vi "Update ROI waveform cursor snap selector.vi"(4 "Reset selection to the first element":bool, 8 "error in (no error)":errorcluster) -> (0 "error out":errorcluster)   [LabVIEW 2020]
uses:
  Global variables/gl_Functional Imaging-Global variables.vi
  <userlib>/_OpenG.lib/array/array.llb/Conditional Auto-Indexing Tunnel (String)__ogtk.vi
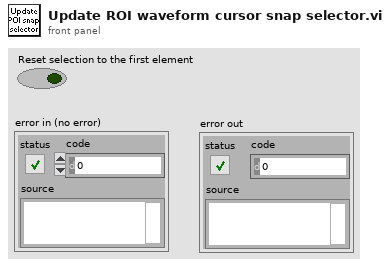
[diagram p1: front panel]
types:
  T1 = typedef "Functional Imging UI Refs.ctl" = cluster{"Menu ref":refnum<k9>, "Image control":refnum<vi>, "VI ref":refnum<vi>, "XGrapher":refnum<vi>, "Smoothing":refnum<vi>, "POI Averaging":refnum<vi>, "Normalize":refnum<vi>, "POI data points in each trial":refnum<vi>, "Channel":refnum<vi>, "Experiment data folder path":refnum<vi>, "[ROI vis]":refnum<vi>, "[Groups] visbl":T2, "Group Name":refnum<vi>, "POI index":refnum<vi>, "Trial No.":refnum<vi>, "Intensity Zoom":refnum<vi>, "Trial Cursor Enabled":refnum<vi>, "Number of Trials (ind 1)":refnum<vi>, "Number of Trials (ind 2)":refnum<vi>, "MiniScans Available":refnum<vi>, "POI Available":refnum<vi>, "Defer graph updates":refnum<vi>, "Waveform selector":refnum<vi>, "#of selected POI":refnum<vi>, "#of selected MiniScans":refnum<vi>, "#of selected groups":refnum<vi>, "Max Z-Projection":refnum<vi>, "Z-Plane Selector":refnum<vi>, "Index of miniscan point to visualise":refnum<vi>, "ROI vis. mode":refnum<vi>, "Total # of points":refnum<vi>, "Index of group clicked on":refnum<vi>, "Pane 1":refnum<vi>, "Pane 2":refnum<vi>, "Pane 3":refnum<vi>, "Pane 4":refnum<vi>, "Pane 5":refnum<vi>, "Pane 6":refnum<vi>, "Deselect all ROI":refnum<vi>, "Deselect all groups":refnum<vi>}
  T2 = typedef "Groups array referecne.ctl" = refnum<vi>
  T3 = typedef "ROI selector array-ROI vis.ctl" = T4[]
  T4 = typedef "Interface-ROI selection cluster.ctl" = cluster{"ROI number":i32, "ROI ID":T5, "Visibility":bool}
  T5 = typedef "ROI ID Enum.ctl" = enum16{"Point", "MiniScan", "Comp. MiniScan", "Rectangle", "Comp. volume", "Arb. plane point", "None"}
  T6 = typedef "Group sel cluster.ctl" = cluster{"Group number":string, "Group Name":string, "Visibility":bool, "Highlight":bool}
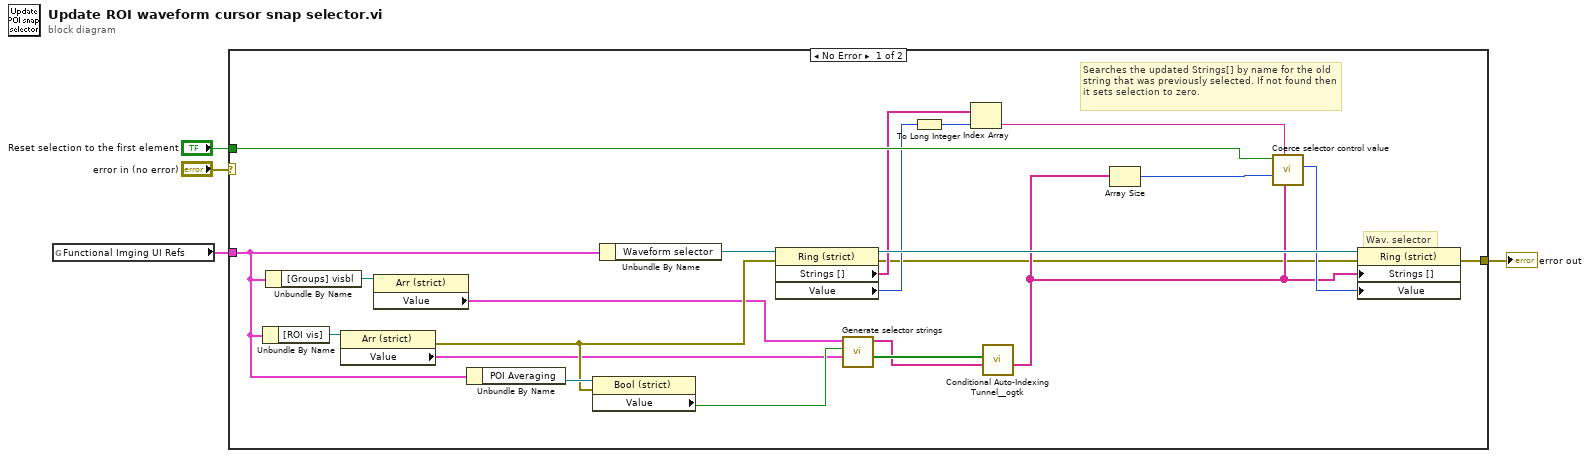
[diagram p0: block diagram]
diagram:
  n1 = global read "gl_Functional Imaging-Global variables.vi" "Functional Imging UI Refs"() -> (w1:T1)
  n2 = case shown="No Error" "error in (no error)" {
    selector: "error in (no error)" -> [_ w27]
    tunnel: [w14 w27] -> w4
    tunnel: w1 -> [w11 _]
    tunnel: "Reset selection to the first element" -> [w19 _]
    frame No Error {
      # "Searches the updated Strings[] by name for the old string that was previously selected. If not found then it sets selection to zero."
      # "Wav. selector"
      # "Updates the POI waveform selector control"
      n3 = Unbundle By Name(w11) -> ("[ROI vis]"=w20:refnum<vi>)
      n4 = Unbundle By Name(w11) -> ("[Groups] visbl"=w12:T2)
      n5 = property on="Property Node" class="Arr (strict)"(reference=w20) -> (error out=w13:errorcluster, "Value"=w10:T3)  [unwired: 1 in, 1 out]
      n6 = property on="Property Node" class="Arr (strict)"(reference=w12) -> ("Value"=w9:T6[])  [unwired: 1 in, 2 out]
      n7 = Unbundle By Name(w11) -> ("POI Averaging"=w24:refnum<vi>)
      n8 = property on="Property Node" class="Bool (strict)"(reference=w24, error in=w13) -> ("Value"=w23:bool)  [unwired: 2 out]
      n9 = Unbundle By Name(w11) -> ("Waveform selector"=w25:refnum<vi>)
      n10 = property on="Property Node" class="Ring (strict)"(reference=w25, error in=w13) -> (reference out=w26:refnum<vi>, error out=w5:errorcluster, "Strings []"=w18:string[], "Value"=w17:u16)
      n11 = call "Generate selector strings.vi"("[POI#] or [MiniScan#]"=w10, "POI Averaged"=w23, "Groups"=w9) -> ("[Visibility]"=w8:bool[], "All group and ROI Strings[]"=w7:string[])  [unwired: 7 in]
      n12 = To Long Integer(number=w17) -> (32bit integer=w16:i32)
      n13 = Index Array(array=w18, index=w16) -> (element=w15:string)
      n14 = call-poly <userlib>:"Conditional Auto-Indexing Tunnel__ogtk.vi"("Array in"=w7, "Elements to keep"=w8) -> ("Filtered Array out"=w6:string[])  [unwired: 5 in]
      n15 = Array Size(array=w6) -> (size(s)=w22:i32)
      n16 = call "Coerce selector control value.vi"("New strings[]"=w6, "String of currently selected item"=w15, "#of selected ROI"=w22, "Set selection to index 0"=w19) -> ("Selection index out"=w21:u16)  [unwired: 7 in]
      n17 = property on="Property Node" class="Ring (strict)"(reference=w26, error in=w5, "Strings []"=w6, "Value"=w21) -> (error out=w14:errorcluster)  [unwired: 1 out]
    }
    frame Error {
    }
  }
  "error out" <- w4
